vi "Drive Controller.vi"(8 "error in":errorcluster) -> ()   [LabVIEW 2019]
doc: "This VI executes continuously carrying out the current operation and responding to updates or new operation requests. It will often contain the timing or control code that is difficult to place directly in TeleOp. This VI generally opens all sensors and motors and isolates the rest of the robot code from knowing implementation details of how the operations are carried out."
uses:
  <vilib>/Rock Robotics/WPI/Framework/Completion Status.ctl
  Drive Setpoints.ctl
  Drive Operations.ctl
  <vilib>/Rock Robotics/WPI/SafetyOutput/WPI_SafetyOutputConfigMenu.ctl
  <vilib>/Rock Robotics/SystemInterfaces/DIO/FPGA_DIOChannel.ctl
  <vilib>/Rock Robotics/WPI/Counter/WPI_CounterEdgeLevel.ctl
  <vilib>/Rock Robotics/WPI/Encoder/WPI_EncoderType.ctl
  <vilib>/Rock Robotics/WPI/Counter/WPI_CounterDigitalInputToDigitalSource.vi
  <vilib>/Rock Robotics/WPI/RobotDrive/WPI_RobotDriveOpen2MotorWithExistingMotors.vi
panel:
  in  "Interactive Values":T1
  in  "Buttons":cluster{"Execute Cmd":bool, "Abort Cmd":bool}
  out "Command Timing":cluster{"Start Time (ms)":u32, "Iterations":i32}
  out "Status":T3
  out "Setpoints":T4(graph)
  out "Current\nCmd":string
  # "Tip: The graph shows the motor setpoints. It may also be helpful to observe inputs and sensor values.\nYou may also want to display tuning or debugging controls."
  # "Interactive Command: You may fill in the settings for a command\nand schedule it with the Execute button. You can observe and abort\nany command while fine tuning the code for the controller."
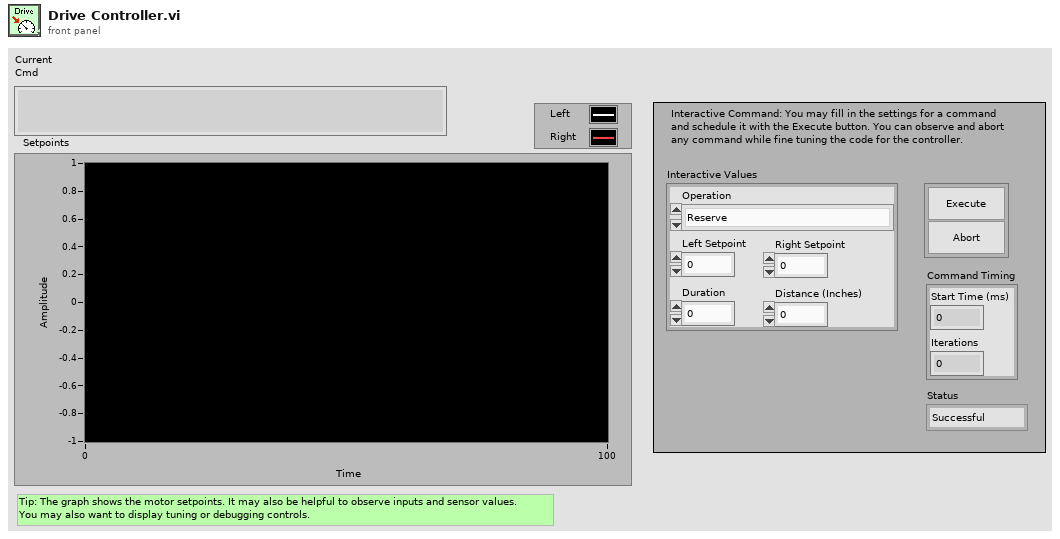
[diagram p1: front panel]
types:
  T1 = typedef "Drive Setpoints.ctl" = cluster{"Operation":T2, "Left Setpoint":dbl, "Right Setpoint":dbl, "Duration":dbl, "Distance (Inches)":dbl}
  T2 = typedef "Drive Operations.ctl" = enum16{"Reserve", "Read Current", "Immediate", "Drive for Time", "Drive for Distance"}
  T3 = typedef "Completion Status.ctl" = enum16{"Successful", "Aborted", "Incomplete"}
  T4 = cluster{"Left Setpoint":dbl, "Right Setpoint":dbl}
  T5 = typedef "WPI_EncoderType.ctl" = enum16{"1x", "2x", "4x"}
  T6 = typedef "WPI_CounterEdgeLevel.ctl" = enum16{"Active Low", "Active High", "Falling Edge", "Rising Edge"}
  T7 = typedef "FPGA_DIOChannel.ctl" = enum8{"DIO 0", "DIO 1", "DIO 2", "DIO 3", "DIO 4", "DIO 5", "DIO 6", "DIO 7", "DIO 8", "DIO 9", "DIO MXP 0", "DIO MXP 1", "DIO MXP 2", "DIO MXP 3", "DIO MXP 4", "DIO MXP 5", "DIO MXP 6", "DIO MXP 7", "DIO MXP 8", "DIO MXP 9", "DIO MXP 10", "DIO MXP 11", "DIO MXP 12", "DIO MXP 13", "DIO MXP 14", "DIO MXP 15", "SPI Port CS1", "SPI Port CS2", "SPI Port CS3", "SPI Port MISO", "SPI Port MOSI", "Invalid"}
  T8 = typedef "WPI_SafetyOutputConfigMenu.ctl" = enum16{"Enable", "Disable"}
  T9 = typedef "WPI_MotorControlDeviceRef.ctl" = cluster{"DeviceStatus":errorcluster, "Type":T10, "PWM":cluster{"PWM Channel":T11, "DeadBand":T12}, "CAN":cluster{"Device Number":u8, "SetOutput VI Ref":variant, "GetOutput VI Ref":variant, "Enable VI Ref":variant, "Disable VI Ref":variant, "Data":variant}, "Invert":bool, "DIO PWM":cluster{"PWM \"Enable\" Channel":T11, "DIOChannel":T7, "PWM Rate":dbl}}
  T10 = typedef "WPI_MotorControlType.ctl" = enum16{"PWM", "CAN", "DIO PWM"}
  T11 = typedef "FPGA_DIOPWMChannel.ctl" = enum8{"PWM 0", "PWM 1", "PWM 2", "PWM 3", "PWM 4", "PWM 5", "PWM 6", "PWM 7", "PWM 8", "PWM 9", "PWM MXP 0", "PWM MXP 1", "PWM MXP 2", "PWM MXP 3", "PWM MXP 4", "PWM MXP 5", "PWM MXP 6", "PWM MXP 7", "PWM MXP 8", "PWM MXP 9", "Invalid"}
  T12 = typedef "WPI_PWMDeadband.ctl" = cluster{"Name":string, "maxPositivePwm":i32, "minPositivePwm":i32, "centerPwm":i32, "maxNegativePwm":i32, "minNegativePwm":i32, "angularRange":u16}
  T13 = typedef "WPI_DigitalInputDevRef.ctl" = cluster{"DevStatus":errorcluster, "DIO Channel":T7}
  T14 = typedef "FPGA_CounterEncoderSourceConvertionLVSourceType.ctl" = cluster{"DevStatus":errorcluster, "AnalogTriggerMode?":bool, "DigitalMode":cluster{"DIO Channel":T15}, "AnalogTriggerMode":cluster{"AnalogTriggerIndex":T16, "OutputType":T17}}
  T15 = typedef "FPGA_DIODigitalSourceChannel.ctl" = enum8{"DIO 0", "DIO 1", "DIO 2", "DIO 3", "DIO 4", "DIO 5", "DIO 6", "DIO 7", "DIO 8", "DIO 9", "DIO MXP 0", "DIO MXP 1", "DIO MXP 2", "DIO MXP 3", "DIO MXP 4", "DIO MXP 5", "DIO MXP 6", "DIO MXP 7", "DIO MXP 8", "DIO MXP 9", "DIO MXP 10", "DIO MXP 11", "DIO MXP 12", "DIO MXP 13", "DIO MXP 14", "DIO MXP 15", "SPI Port CS1", "SPI Port CS2", "SPI Port CS3", "SPI Port MISO", "SPI Port MOSI", "Disabled"}
  T16 = typedef "FPGA_AnalogTriggerIndex.ctl" = enum8{"Trig 0", "Trig 1", "Trig 2", "Trig 3", "Trig 4", "Trig 5", "Trig 6", "Trig 7", "Invalid"}
  T17 = typedef "FPGA_AnalogTriggerOutType.ctl" = enum16{"InWindow", "TriggerState", "Rising", "Falling"}
  T18 = typedef "WPI_EncoderDevRef.ctl" = cluster{"DevStatus":errorcluster, "EncoderIndex":T19, "CounterIndex":T20, "DistancePerCount":dbl, "Decoding Type":T5}
  T19 = typedef "FPGA_EncoderIdx.ctl" = enum8{"Enc 0", "Enc 1", "Enc 2", "Enc 3", "Enc 4", "Enc 5", "Enc 6", "Enc 7", "Invalid"}
  T20 = typedef "FPGA_CounterCtrSystemIndex.ctl" = enum8{"Ctr 0", "Ctr 1", "Ctr 2", "Ctr 3", "Ctr 4", "Ctr 5", "Ctr 6", "Ctr 7", "Invalid"}
  T21 = typedef "WPI_RobotDriveDevRef.ctl" = cluster{"DevStatus":errorcluster, "Motors[]":T9[], "Square Inputs":bool, "Max Output":dbl}
  T22 = typedef "Command Status Info.ctl" = cluster{"Name":string, "Status":T3, "notifier out":T23}
  T23 = typedef "Completion Notifier.ctl" = refnum<notifier>
  T24 = cluster{"SubSystem Data":T1, cluster{"Start Time (ms)":u32, "Iterations":i32}, cluster{"Command Info":T22, "Description":string, "Default Command":T1, "queue out":refnum<queue>, "Subsystem Name":string}}
  T25 = cluster{"SubSystem Data":T1, cluster{"Start Time (ms)":u32, "Iterations":i32}, "Default Command Arguments":cluster{"Command Info":T22, "Description":string, "Default Command":T1, "queue out":refnum<queue>, "Subsystem Name":string}}
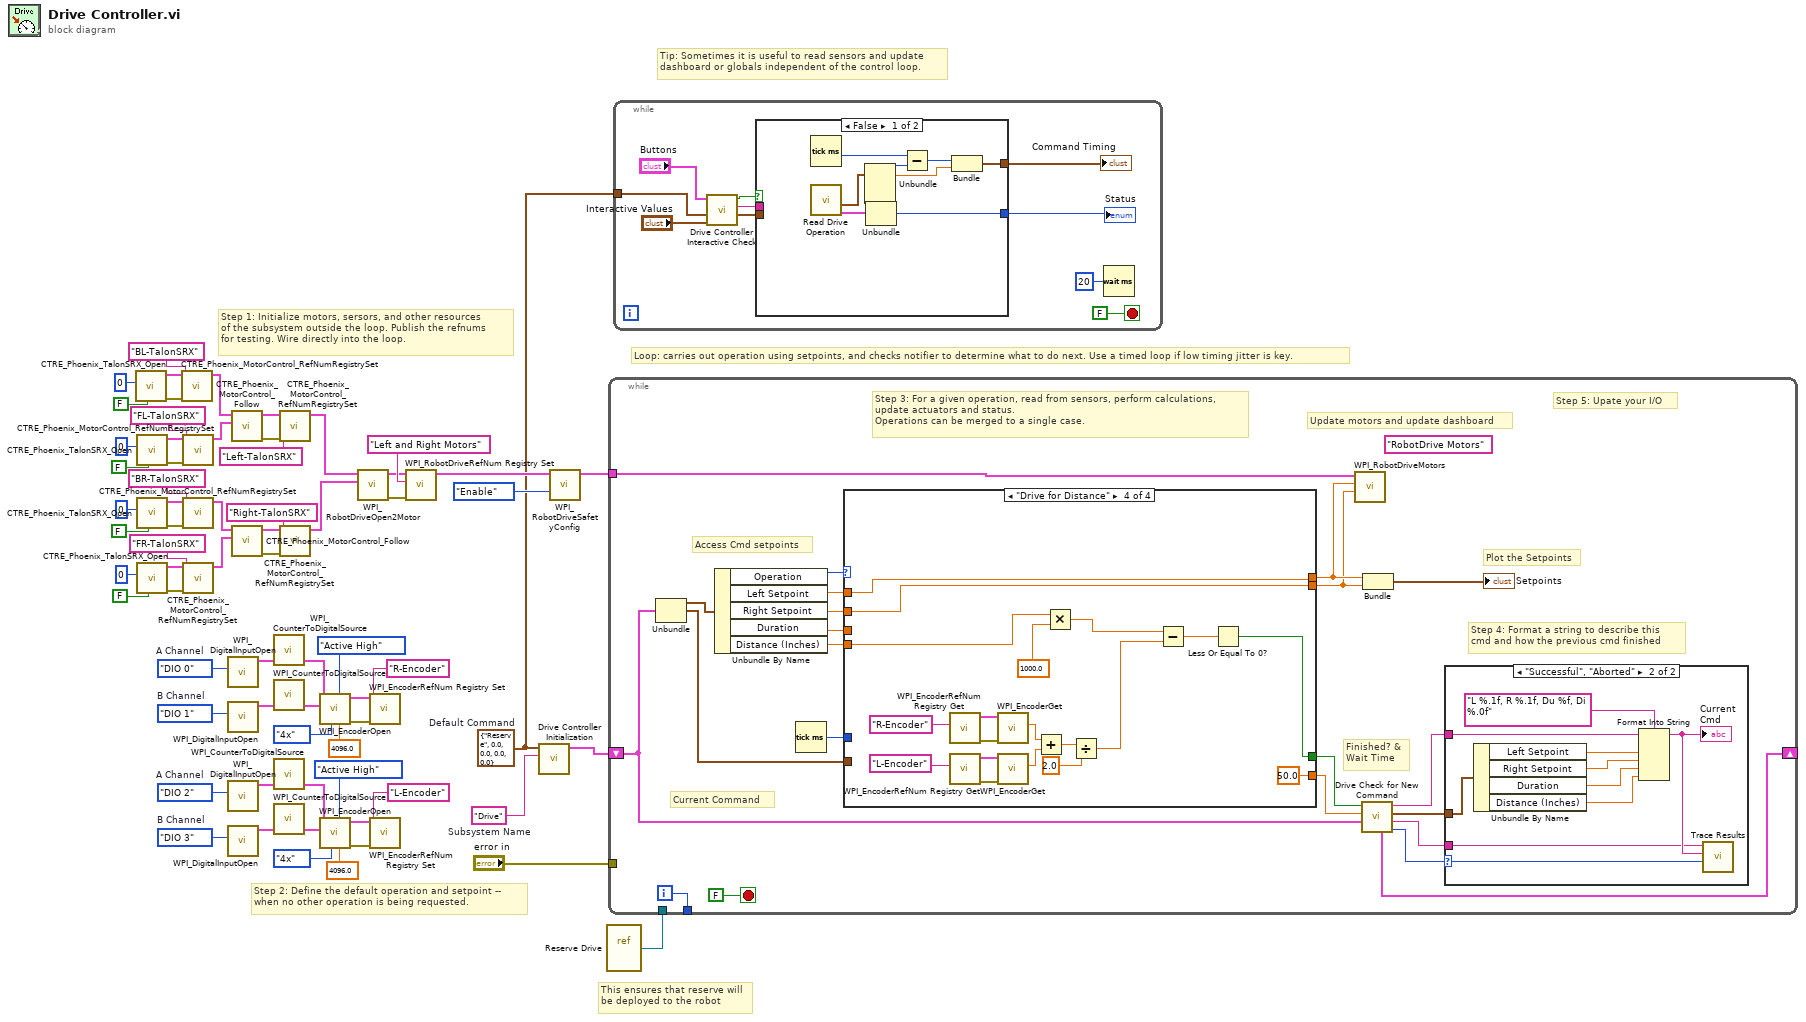
[diagram p0: block diagram]
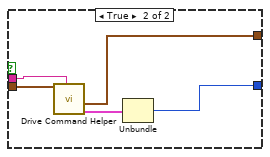
[diagram p2: hidden frame]
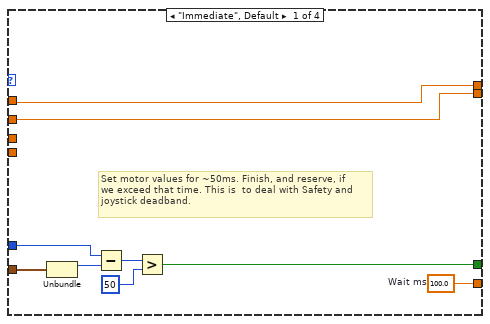
[diagram p4: hidden frame]
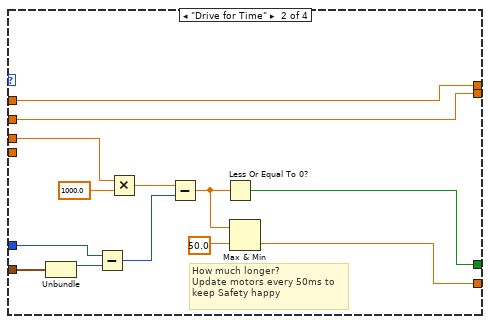
[diagram p5: hidden frame]
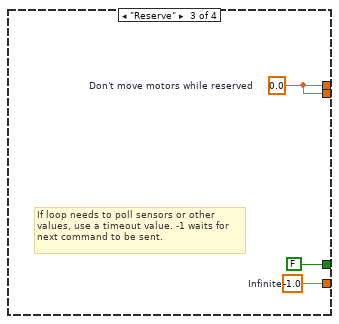
[diagram p6: hidden frame]
diagram:
  w49 = FPGA_DIOChannel."DIO 3"  # B Channel
  w48 = FPGA_DIOChannel."DIO 2"  # A Channel
  w58 = FPGA_DIOChannel."DIO 1"  # B Channel
  w57 = FPGA_DIOChannel."DIO 0"  # A Channel
  w59 = T1 {"Operation"=enum."Reserve", "Left Setpoint"=0.0, "Right Setpoint"=0.0, "Duration"=0.0, "Distance (Inches)"=0.0}  # Default Command
  w67 = "Drive"  # Subsystem Name
  # "This ensures that reserve will\nbe deployed to the robot"
  # "Tip: Sometimes it is useful to read sensors and update\ndashboard or globals independent of the control loop."
  # "Step 2: Define the default operation and setpoint --\nwhen no other operation is being requested."
  # "Step 1: Initialize motors, sersors, and other resources\nof the subsystem outside the loop. Publish the refnums\nfor testing. Wire directly into the loop."
  # "Loop: carries out operation using setpoints, and checks notifier to determine what to do next. Use a timed loop if low timing jitter is key."
  n1 = call <vilib>:"CTRE_Phoenix_TalonSRX_Open.vi"("Invert"=FALSE, "Device Number"=u8 0) -> ("error out"=w32:errorcluster, "CAN Talon SRX Ref"=w31:T9)  [unwired: 8 in]
  n2 = call <vilib>:"CTRE_Phoenix_TalonSRX_Open.vi"("Invert"=FALSE, "Device Number"=u8 0) -> ("error out"=w28:errorcluster, "CAN Talon SRX Ref"=w27:T9)  [unwired: 8 in]
  n3 = call <vilib>:"CTRE_Phoenix_TalonSRX_Open.vi"("Invert"=FALSE, "Device Number"=u8 0) -> ("error out"=w24:errorcluster, "CAN Talon SRX Ref"=w23:T9)  [unwired: 8 in]
  n4 = call <vilib>:"CTRE_Phoenix_TalonSRX_Open.vi"("Invert"=FALSE, "Device Number"=u8 0) -> ("error out"=w20:errorcluster, "CAN Talon SRX Ref"=w19:T9)  [unwired: 8 in]
  n5 = call <vilib>:"CTRE_Phoenix_MotorControl_RefNumRegistrySet.vi"("error in (no error)"=w32, "refnum name"="BL-TalonSRX", "PhoenixMotorControlDevRef"=w31) -> ("PhoenixMotorControlDevRef"=w15:T9)  [unwired: 7 in, 1 out]
  n6 = call <vilib>:"CTRE_Phoenix_MotorControl_RefNumRegistrySet.vi"("error in (no error)"=w28, "refnum name"="FL-TalonSRX", "PhoenixMotorControlDevRef"=w27) -> ("PhoenixMotorControlDevRef"=w16:T9)  [unwired: 7 in, 1 out]
  n7 = call <vilib>:"CTRE_Phoenix_MotorControl_RefNumRegistrySet.vi"("error in (no error)"=w24, "refnum name"="BR-TalonSRX", "PhoenixMotorControlDevRef"=w23) -> ("PhoenixMotorControlDevRef"=w8:T9)  [unwired: 7 in, 1 out]
  n8 = call <vilib>:"CTRE_Phoenix_MotorControl_RefNumRegistrySet.vi"("error in (no error)"=w20, "refnum name"="FR-TalonSRX", "PhoenixMotorControlDevRef"=w19) -> ("PhoenixMotorControlDevRef"=w7:T9)  [unwired: 7 in, 1 out]
  n9 = call <vilib>:"WPI_DigitalInputOpen.vi"("DIO Channel"=w57) -> ("DigitalInputDevRef"=w54:T13)  [unwired: 1 in, 9 out]
  n10 = call <vilib>:"WPI_DigitalInputOpen.vi"("DIO Channel"=w58) -> ("DigitalInputDevRef"=w55:T13)  [unwired: 1 in, 9 out]
  n11 = call <vilib>:"WPI_DigitalInputOpen.vi"("DIO Channel"=w48) -> ("DigitalInputDevRef"=w45:T13)  [unwired: 1 in, 9 out]
  n12 = call <vilib>:"WPI_DigitalInputOpen.vi"("DIO Channel"=w49) -> ("DigitalInputDevRef"=w46:T13)  [unwired: 1 in, 9 out]
  n13 = call <vilib>:"CTRE_Phoenix_MotorControl_Follow.vi"("Master Controller to Follow"=w16, "PhoenixMotorControlDevRef"=w15) -> ("error out"=w14:errorcluster, "PhoenixMotorControlDevRef"=w13:T9)  [unwired: 8 in]
  n14 = call <vilib>:"CTRE_Phoenix_MotorControl_Follow.vi"("Master Controller to Follow"=w7, "PhoenixMotorControlDevRef"=w8) -> ("error out"=w12:errorcluster, "PhoenixMotorControlDevRef"=w11:T9)  [unwired: 8 in]
  n15 = call-poly <vilib>:"WPI_CounterToDigitalSource.vi"("DigitalInputDevRef"=w54) -> ("Digital Source"=w53:T14)  [unwired: 6 out]
  n16 = call-poly <vilib>:"WPI_CounterToDigitalSource.vi"("DigitalInputDevRef"=w55) -> ("Digital Source"=w56:T14)  [unwired: 6 out]
  n17 = call-poly <vilib>:"WPI_CounterToDigitalSource.vi"("DigitalInputDevRef"=w45) -> ("Digital Source"=w44:T14)  [unwired: 6 out]
  n18 = call-poly <vilib>:"WPI_CounterToDigitalSource.vi"("DigitalInputDevRef"=w46) -> ("Digital Source"=w47:T14)  [unwired: 6 out]
  n19 = call <vilib>:"CTRE_Phoenix_MotorControl_RefNumRegistrySet.vi"("error in (no error)"=w14, "refnum name"="Left-TalonSRX", "PhoenixMotorControlDevRef"=w13) -> ("PhoenixMotorControlDevRef"=w10:T9)  [unwired: 7 in, 1 out]
  n20 = call <vilib>:"CTRE_Phoenix_MotorControl_RefNumRegistrySet.vi"("error in (no error)"=w12, "refnum name"="Right-TalonSRX", "PhoenixMotorControlDevRef"=w11) -> ("PhoenixMotorControlDevRef"=w9:T9)  [unwired: 7 in, 1 out]
  n21 = call <vilib>:"WPI_EncoderOpen.vi"("DistancePerCount"=4096.0, "External Reset Trigger"=WPI_CounterEdgeLevel."Active High", "Decoding Type"=WPI_EncoderType."4x", "BSource"=w56, "ASource"=w53) -> ("error out"=w52:errorcluster, "EncoderDevRef"=w51:T18)  [unwired: 3 in, 2 out]
  n22 = call <vilib>:"WPI_EncoderOpen.vi"("DistancePerCount"=4096.0, "External Reset Trigger"=WPI_CounterEdgeLevel."Active High", "Decoding Type"=WPI_EncoderType."4x", "BSource"=w47, "ASource"=w44) -> ("error out"=w43:errorcluster, "EncoderDevRef"=w42:T18)  [unwired: 3 in, 2 out]
  n23 = call-poly <vilib>:"WPI_RobotDriveOpen2Motor.vi"("Right Motor Dev Ref"=w9, "Left Motor Dev Ref"=w10) -> ("error out"=w34:errorcluster, "RobotDriveDevRef"=w33:T21)  [unwired: 8 in]
  n24 = call <vilib>:"WPI_EncoderRefNum Registry Set.vi"("error in (no error)"=w52, "refnum name"="R-Encoder", "EncoderDevRef"=w51) -> ()  [unwired: 7 in, 2 out]
  n25 = call <vilib>:"WPI_EncoderRefNum Registry Set.vi"("error in (no error)"=w43, "refnum name"="L-Encoder", "EncoderDevRef"=w42) -> ()  [unwired: 7 in, 2 out]
  n26 = call <vilib>:"WPI_RobotDriveRefNum Registry Set.vi"("error in (no error)"=w34, "refnum name"="Left and Right Motors", "RobotDriveDevRef"=w33) -> ("RobotDriveDevRef"=w65:T21)  [unwired: 1 in, 7 out]
  n27 = call "Drive Controller Initialization.vi"("Subsystem Name"=w67, "Default Command"=w59) -> ("Current Command"=w61:T24)  [unwired: 9 in]
  n28 = call <vilib>:"WPI_RobotDriveSafetyConfig.vi"("mode"=WPI_SafetyOutputConfigMenu."Enable", "RobotDriveDevRef"=w65) -> ("RobotDriveDevRef"=w63:T21)  [unwired: 8 in, 1 out]
  n29 = vi-ref "Reserve Drive.vi"() -> (w60:refnum<vi>)
  n30 = while {
    shift-right: [w71] -> _
    shift-left: w61 -> [w72]
    tunnel: [w88] -> _
    tunnel: w63 -> [w86]
    tunnel: "error in" -> [_]
    tunnel: w60 -> [_]
    i -> [w88]
    stop <- FALSE stop-if-true
    (unwired) "RobotDrive Motors" ("Name")
    # "Step 5: Upate your I/O"
    # "Step 4: Format a string to describe this\ncmd and how the previous cmd finished"
    # "Current Command"
    # "Update motors and update dashboard"
    # "Plot the Setpoints"
    # "Access Cmd setpoints"
    # "Finished? &\nWait Time"
    # "Step 3: For a given operation, read from sensors, perform calculations,\nupdate actuators and status.\nOperations can be merged to a single case."
    n31 = Unbundle(w72) -> ("SubSystem Data"=w85:T1, w73:cluster{"Start Time (ms)":u32, "Iterations":i32})  [unwired: 1 out]
    n32 = Unbundle By Name(w85) -> ("Operation"=w84:T2, "Left Setpoint"=w83:dbl, "Right Setpoint"=w82:dbl, "Duration"=w81:dbl, "Distance (Inches)"=w70:dbl)
    n33 = Tick Count (ms)() -> (millisecond timer value=w80:u32)
    n34 = case shown="\"Drive for Distance\"" w84 {
      tunnel: [w108 w109 w124 50.0 ("Infinite")] -> w78
      tunnel: [w101 w116 FALSE ("ignore previous (F)") w128] -> w77
      tunnel: w73 -> [w100 w118 _ _]
      tunnel: [w107 w115 w122 w125] -> w69
      tunnel: [w106 w114 w122 w126] -> w68
      tunnel: w83 -> [w107 w115 _ w125]
      tunnel: w82 -> [w106 w114 _ w126]
      tunnel: w81 -> [_ w113 _ _]
      tunnel: w80 -> [w102 w112 _ _]
      tunnel: w70 -> [_ _ _ w140]
      frame "Immediate", Default {
        w108 = 100.0  # Wait ms
        # "Set motor values for ~50ms. Finish, and reserve, if\nwe exceed that time. This is  to deal with Safety and\njoystick deadband."
        n35 = Unbundle(w100) -> ("Start Time (ms)"=w103:u32)  [unwired: 1 out]
        n36 = Subtract(x=w102, y=w103) -> (x-y=w104:u32)
        n37 = Greater?(x=w104, y=u8 50 ("Left Motor")) -> (0:w101:bool)
      }
      frame "Drive for Time" {
        # "How much longer?\nUpdate motors every 50ms to\nkeep Safety happy"
        n38 = Unbundle(w118) -> ("Start Time (ms)"=w117:u32)  [unwired: 1 out]
        n39 = Subtract(x=w112, y=w117) -> (x-y=w121:u32)
        n40 = Multiply(x=w113, y=1000.0) -> (x*y=w120:dbl)
        n41 = Subtract(x=w120, y=w121) -> (x-y=w111:dbl)
        n42 = Less Or Equal To 0?(x=w111) -> (x <= 0?=w116:bool)
        n43 = Max & Min(x=w111, y=50.0) -> (min(x,y)=w109:dbl)  [unwired: 1 out]
      }
      frame "Reserve" {
        w122 = 0.0  # Don't move motors while reserved
        w124 = -1.0  # Infinite
        # "If loop needs to poll sensors or other\nvalues, use a timeout value. -1 waits for\nnext command to be sent."
      }
      frame "Drive for Distance" {
        n44 = call <vilib>:"WPI_EncoderRefNum Registry Get.vi"("refnum name"="R-Encoder") -> ("error out"=w139:errorcluster, "EncoderDevRef"=w138:T18)  [unwired: 9 in]
        n45 = call <vilib>:"WPI_EncoderRefNum Registry Get.vi"("refnum name"="L-Encoder") -> ("error out"=w136:errorcluster, "EncoderDevRef"=w137:T18)  [unwired: 9 in]
        n46 = call <vilib>:"WPI_EncoderGet.vi"("error in (no error)"=w139, "EncoderDevRef"=w138) -> ("Distance"=w133:dbl)  [unwired: 4 in, 5 out]
        n47 = call <vilib>:"WPI_EncoderGet.vi"("error in (no error)"=w136, "EncoderDevRef"=w137) -> ("Distance"=w132:dbl)  [unwired: 4 in, 5 out]
        n48 = Add(x=w133, y=w132) -> (x+y=w131:dbl)
        n49 = Multiply(x=w140, y=1000.0) -> (x*y=w142:dbl)
        n50 = Divide(x=w131, y=2.0) -> (x/y=w129:dbl)
        n51 = Subtract(x=w142, y=w129) -> (x-y=w143:dbl)
        n52 = Less Or Equal To 0?(x=w143) -> (x <= 0?=w128:bool)
      }
    }
    n53 = call <vilib>:"WPI_RobotDriveMotors.vi"("RightSpeed"=w68, "LeftSpeed"=w69, "RobotDriveDevRef"=w86) -> ()  [unwired: 1 in, 8 out]
    n54 = call "Drive Check for New Command.vi"("input cluster"=w72, "Wait time (ms)"=w78, "Finished?"=w77) -> ("Completion"=w79:T3, "Subsystem Name"=w74:string, "Current Command"=w75:T1, "Initial Trace String"=w76:string, "Next Command"=w71:T25)  [unwired: 4 in]
    n55 = Bundle("Left Setpoint"=w69, "Right Setpoint"=w68) -> (→"Setpoints":T4)  [unwired: 1 in]
    n56 = case shown="\"Successful\", \"Aborted\"" w79 {
      selector: w79 -> [_ w99]
      tunnel: w76 -> [_ w94]
      tunnel: w75 -> [_ w95]
      tunnel: w74 -> [_ w91]
      frame "Incomplete", Default {
        # "Continuing current command"
      }
      frame "Successful", "Aborted" {
        # "Report and setup for next command"
        n57 = Unbundle By Name(w95) -> ("Left Setpoint"=w97:dbl, "Right Setpoint"=w98:dbl, "Duration"=w92:dbl, "Distance (Inches)"=w90:dbl)
        n58 = Format Into String(format string="L %.1f, R %.1f, Du %f, Di %.0f", initial string=w94, w97, w98, w92, w90) -> (resulting string=w93:string)  [unwired: 1 in, 1 out]
        "Current\nCmd" <- w93
        n59 = call <vilib>:"Trace Results.vi"("Status of previous command"=w99, "Description"=w93, "Subsystem"=w91) -> ()  [unwired: 9 in]
      }
    }
  }
  n60 = while {
    tunnel: w59 -> [w145]
    stop <- FALSE stop-if-true
    n61 = call "Drive Controller Interactive Check.vi"("Interactive Command In"="Interactive Values", "Default Command"=w145, "Buttons"="Buttons") -> ("Interactive Command Out"=w147:T1, "Trace String"=w148:string, "Schedule"=w149:bool)  [unwired: 6 in]
    n62 = case shown="False" w149 {
      tunnel: [w158 w166] -> w150
      tunnel: [w157 w162] -> w151
      tunnel: w148 -> [_ w164]
      tunnel: w147 -> [_ w163]
      frame False {
        n63 = Tick Count (ms)() -> (millisecond timer value=w161:u32)
        n64 = call "Read Drive Operation.vi"() -> ("Command Info"=w155:T22, "SubSystem Data"=w154:T1)  [unwired: 9 in, 1 out]
        n65 = Unbundle(w154) -> ("Operation"=w159:T2, "Left Setpoint"=w156:dbl)  [unwired: 3 out]
        n66 = Unbundle(w155) -> ("Status"=w158:T3)  [unwired: 2 out]
        n67 = Subtract(x=w161, y=w159) -> (x-y=w160:u32)
        n68 = Bundle(w160, "Left Setpoint"=w156) -> (w157:cluster{u32, "Left Setpoint":dbl})  [unwired: 1 in]
      }
      frame True {
        n69 = call "Drive Command Helper.vi"("Description"=w164, "SubSystem Data"=w163) -> ("Command Info Out"=w165:T22, "Command Timing"=w162:cluster{"Start Time (ms)":u32, "Iterations":i32})  [unwired: 7 in, 1 out]
        n70 = Unbundle(w165) -> ("Status"=w166:T3)  [unwired: 2 out]
      }
    }
    "Status" <- w150
    "Command Timing" <- w151
    n71 = Wait (ms)(milliseconds to wait=u32 20) -> ()  [unwired: 1 out]
  }
